vi "lm Init.vi"(8 "error in (no error)":errorcluster, 10 "LETypeStr":string, 11 "ComPort":i32) -> (0 "error out":errorcluster, 2 "LETypeStr out":string, 3 "function return":u32)   [LabVIEW 2015, in "LumencorDLL32.lvlib"]
doc: "This function Initializes the Light Engine.. The LE Type is the LE Type Name string. (SPECTRA7, SOLA etc.) in all upper case.\nThe Com port is the com port number to be opened. This is a 0 based number so Com-1 would be 0, Com-2 = 1 etc.\n\nextern \"C\" LUMENCORDLL2B_API HANDLE lmInit(int ComPort, char *LETypeStr);"
uses:
  <userlib>/LumencorDLL32/LumencorDLL32.lvlib
  <userlib>/LumencorDLL32/LumencorDLL32.dll
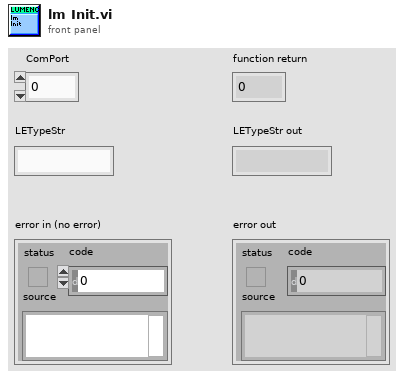
[diagram p1: front panel]
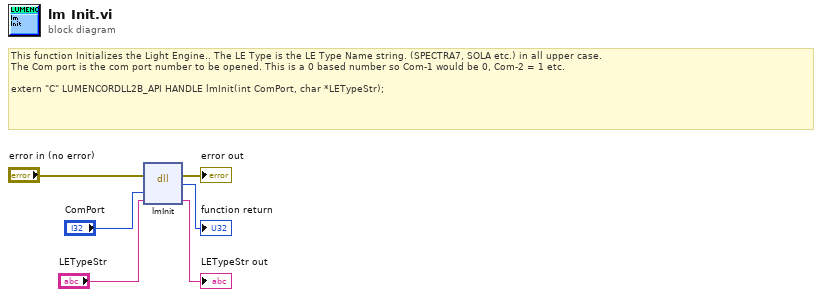
[diagram p0: block diagram]
diagram:
  # "This function Initializes the Light Engine.. The LE Type is the LE Type Name string. (SPECTRA7, SOLA etc.) in all upper case.\nThe Com port is the com port number to be opened. This is a 0 based number so Com-1 would be 0, Com-2 = 1 etc.\n\nextern \"C\" LUMENCORDLL2B_API HANDLE lmInit(int ComPort, char *LETypeStr);"
  n1 = dll-call lib="C:/Program Files (x86)/National Instruments/LabVIEW 2015/user.lib/LumencorDLL32/LumencorDLL32.*" fn="lmInit"(error in="error in (no error)", "ComPort"="ComPort", "LETypeStr"="LETypeStr") -> (error out=→"error out":errorcluster, →"function return":u32, "LETypeStr"=→"LETypeStr out":string)  [unwired: 3 in, 1 out]
